vi "RotateCoordinate (SubVI).vi"(5 "Units":enum16{"mrad", "Radians", "Degrees"}(ring), 7 "Angle":dbl, 8 "error in (no error)":errorcluster, 9 "y":dbl, 10 "x":dbl) -> (0 "error out":errorcluster, 1 "y'":dbl, 2 "x'":dbl)   [LabVIEW 2016]
uses:
  <vilib>/Analysis/coordinate.llb/2D Cartesian Coordinate Rotation (Scalar).vi
  <vilib>/Analysis/NI_AALPro.lvlib
panel:
  out "cos(a)":dbl
  out "sin(a)":dbl
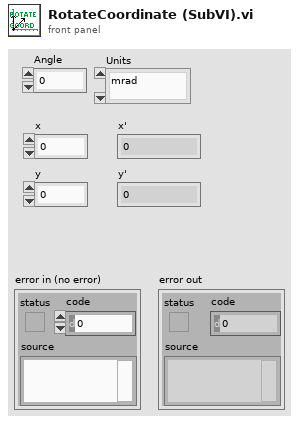
[diagram p1: front panel]
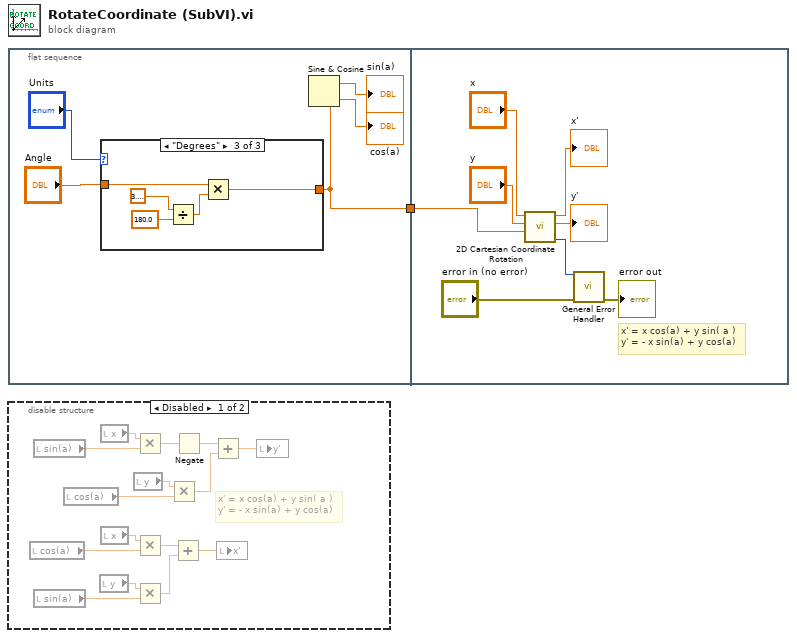
[diagram p0: block diagram]
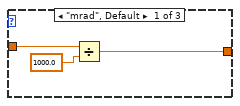
[diagram p3: hidden frame]
diagram:
  n1 = flat-sequence {
    tunnel: [w2] -> w1
    tunnel: w1 -> [w16]
    frame #0 {
      n2 = case shown="\"Degrees\"" "Units" {
        tunnel: "Angle" -> [w9 w10 w13]
        tunnel: [w7 w10 w11] -> w2
        frame "mrad", Default {
          n3 = Divide(x=w9, y=1000.0) -> (x/y=w7:dbl)
        }
        frame "Radians" {
        }
        frame "Degrees" {
          n4 = Divide(x=3.141592653589793, y=180.0) -> (x/y=w14:dbl)
          n5 = Multiply(x=w13, y=w14) -> (x*y=w11:dbl)
        }
      }
      n6 = Sine & Cosine(0:w2) -> (1:→"sin(a)":dbl, 2:→"cos(a)":dbl)
    }
    frame #1 {
      # "x' = x cos(a) + y sin( a )\ny' = - x sin(a) + y cos(a)"
      n7 = call-poly <vilib>:"2D Cartesian Coordinate Rotation.vi"("theta"=w16, "y"="y", "x"="x") -> ("error"=w19:i32, "y out"=→"y'":dbl, "x out"=→"x'":dbl)  [unwired: 6 in]
      n8 = call <vilib>:"General Error Handler.vi"("[error code] (0)"=w19, "error in (no error)"="error in (no error)") -> ("error out"=→"error out":errorcluster)  [unwired: 9 in, 4 out]
    }
  }
  n9 = disable-structure shown="Disabled" {
    frame Disabled {
      # "x' = x cos(a) + y sin( a )\ny' = - x sin(a) + y cos(a)"
      n10 = local read "cos(a)"() -> (w28:dbl)
      n11 = local read "sin(a)"() -> (w33:dbl)
      n12 = local read "sin(a)"() -> (w29:dbl)
      n13 = local read "cos(a)"() -> (w35:dbl)
      n14 = local read "y"() -> (w26:dbl)
      n15 = local read "x"() -> (w32:dbl)
      n16 = local read "x"() -> (w27:dbl)
      n17 = local read "y"() -> (w34:dbl)
      n18 = Multiply(x=w32, y=w33) -> (x*y=w37:dbl)
      n19 = Multiply(x=w27, y=w28) -> (x*y=w30:dbl)
      n20 = Multiply(x=w26, y=w29) -> (x*y=w31:dbl)
      n21 = Multiply(x=w34, y=w35) -> (x*y=w36:dbl)
      n22 = Add(x=w30, y=w31) -> (x+y=w25:dbl)
      n23 = Negate(x=w37) -> (-x=w38:dbl)
      n24 = Add(x=w38, y=w36) -> (x+y=w24:dbl)
      n25 = local write "x'"(w25) -> ()
      n26 = local write "y'"(w24) -> ()
    }
    frame Enabled {
    }
  }
